vi "ButtonStepPlaceNone.vi"(11 "Buttons":bool[](array[boolean])) -> ()   [LabVIEW 2014]
uses:
  Gantry/GantryGlobals.vi
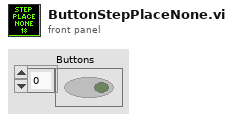
[diagram p1: front panel]
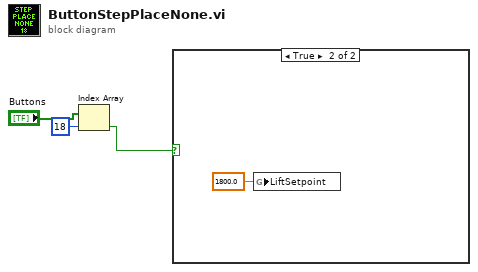
[diagram p0: block diagram]
diagram:
  n1 = Index Array(array="Buttons", index=18) -> (element=w1:bool)
  n2 = case shown="True" w1 {
    frame False {
    }
    frame True {
      n3 = global write "GantryGlobals.vi" "LiftSetpoint"(1800.0 ("LiftSetpoint")) -> ()
    }
  }
